vi "KDH_4th_Ex3Task5_1-24-17.vi"() -> ()   [LabVIEW 2014, in "Harris_MacMaster_4th_LEGORobotics_11-29-16.lvrbt"]
uses:
  Harris_MacMaster_4th_LEGORobotics_11-29-16.lvrbt
  <vilib>/NXT/Dual Mode Library/Sensors/EV3_Ultrasonic_CM.vi
panel:
  out "Error?":bool
  in  "Stop Button":bool
  out "Distance LED":bool
  out "Wall Proximity":string
  in  "Min Distance":dbl
  in  "Max Distance":dbl
  out "Current Distance":dbl
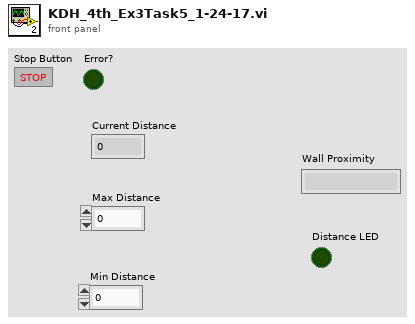
[diagram p1: front panel]
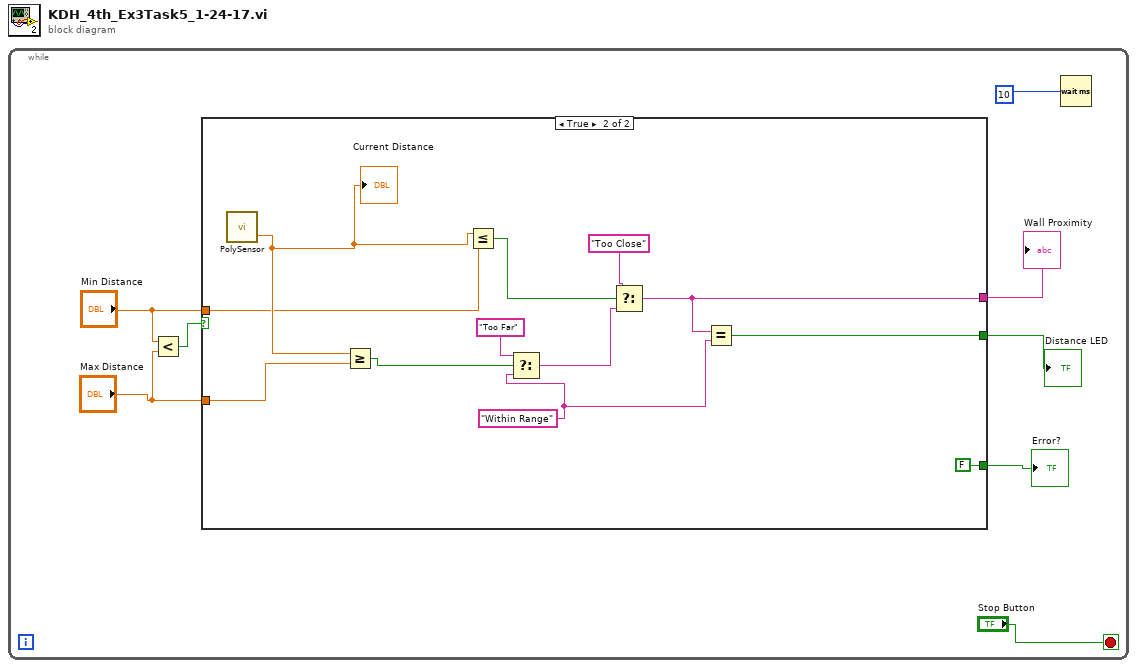
[diagram p0: block diagram]
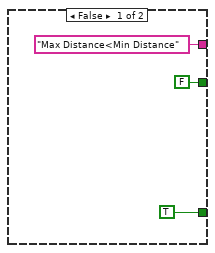
[diagram p2: hidden frame]
diagram:
  n1 = while {
    stop <- "Stop Button" stop-if-true
    n2 = Less?(x="Min Distance", y="Max Distance") -> (x < y?=w6:bool)
    n3 = case shown="True" w6 {
      tunnel: "Max Distance" -> [_ w16]
      tunnel: "Min Distance" -> [_ w15]
      tunnel: ["Max Distance<Min Distance" w14] -> w3
      tunnel: [FALSE w13] -> w2
      tunnel: [TRUE ("Error?") FALSE ("Error?")] -> w1
      frame False {
      }
      frame True {
        w17 = "Within Range"
        n4 = call-poly <vilib>:"PolySensor.vi"() -> ("Centimeters"=w20:sgl)  [unwired: 3 in, 1 out]
        "Current Distance" <- w20
        n5 = Greater Or Equal?(x=w20, y=w16) -> (x >= y?=w23:bool)
        n6 = Less Or Equal?(x=w20, y=w15) -> (x <= y?=w19:bool)
        n7 = Select(t="Too Far", s=w23, f=w17) -> (s? t:f=w18:string)
        n8 = Select(t="Too Close", s=w19, f=w18) -> (s? t:f=w14:string)
        n9 = Equal?(x=w14, y=w17) -> (x = y?=w13:bool)
      }
    }
    "Wall Proximity" <- w3
    "Distance LED" <- w2
    "Error?" <- w1
    n10 = Wait (ms)(milliseconds to wait=u32 10 ("millisecond timer value")) -> ()  [unwired: 1 out]
  }
